vi "144 Swerve Drive 2022.vi"(0 "Joystick X":dbl, 1 "Joystick Y":dbl, 2 "Joystick Z":dbl, 3 "Robot Length(in.)":dbl, 4 "Robot Width(in.)":dbl, 5 "Gyro":dbl, 8 "BL_Steer_Encoder":dbl, 9 "BL PID gains":T1={"proportional gain (Kc)"=0.01, "integral time (Ti, min)"=0.0, "derivative time (Td, min)"=0.0} {"derivative time (Td, min)" format="%.3f"; "integral time (Ti, min)" format="%.3f"; "proportional gain (Kc)" format="%.6f"}, 10 "BR_Steer_Encoder":dbl, 11 "BR PID gains":T1={"proportional gain (Kc)"=0.01, "integral time (Ti, min)"=0.0, "derivative time (Td, min)"=0.0} {"derivative time (Td, min)" format="%.3f"; "integral time (Ti, min)" format="%.3f"; "proportional gain (Kc)" format="%.6f"}, 12 "FL_Steer_Encoder":dbl, 13 "FL PID gains":T1={"proportional gain (Kc)"=0.01, "integral time (Ti, min)"=0.0, "derivative time (Td, min)"=0.0} {"derivative time (Td, min)" format="%.3f"; "integral time (Ti, min)" format="%.3f"; "proportional gain (Kc)" format="%.6f"}, 14 "FR_Steer_Encoder":dbl, 15 "FR PID gains":T1={"proportional gain (Kc)"=0.01, "integral time (Ti, min)"=0.0, "derivative time (Td, min)"=0.0} {"derivative time (Td, min)" format="%.3f"; "integral time (Ti, min)" format="%.3f"; "proportional gain (Kc)" format="%.6f"}) -> (20 "Throttle BL":dbl, 21 "Throttle BR":dbl, 22 "Throttle FL":dbl, 23 "Throttle FR":dbl, 24 "BL_STEER_MOTOR_OUTPUT":dbl, 25 "BR_STEER_MOTOR_OUTPUT":dbl, 26 "FL_STEER_MOTOR_OUTPUT":dbl, 27 "FR_STEER_MOTOR_OUTPUT":dbl)   [LabVIEW 2020]
uses:
  <vilib>/addons/control/pid/pid.llb/PID (DBL).vi
  <vilib>/addons/control/pid/NI_PID_pid.lvlib
panel:
  out "FR_ERROR":dbl
  out "FL_ERROR":dbl
  out "BR_ERROR":dbl
  out "BL_ERROR":dbl
  out "Rotation steering angle BL":dbl
  out "Rotation steering angle FR":dbl
  out "Rotation steering angle FL":dbl
  out "Rotation steering angle BR":dbl
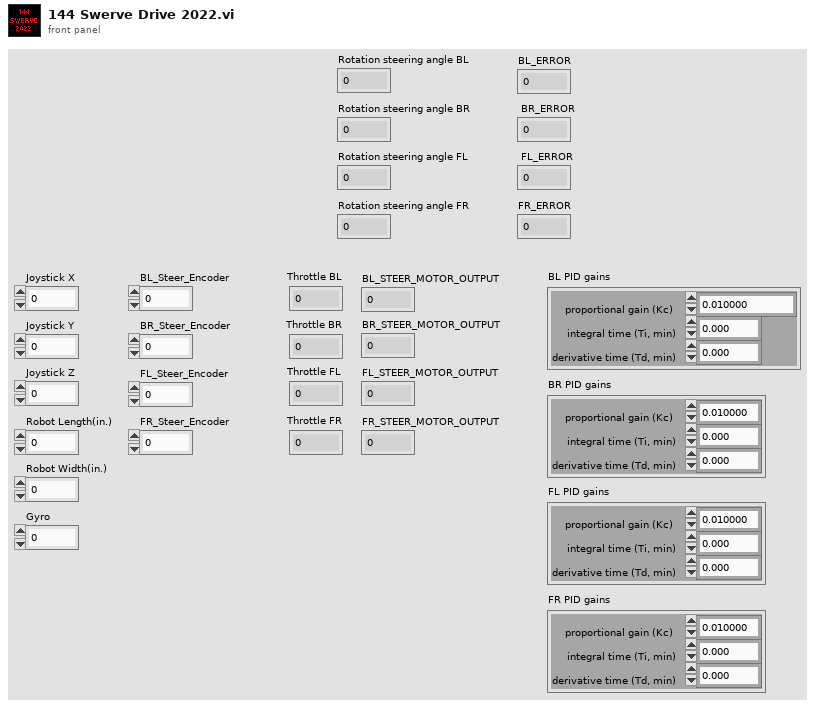
[diagram p1: front panel]
types:
  T1 = cluster{"proportional gain (Kc)":dbl, "integral time (Ti, min)":dbl, "derivative time (Td, min)":dbl}
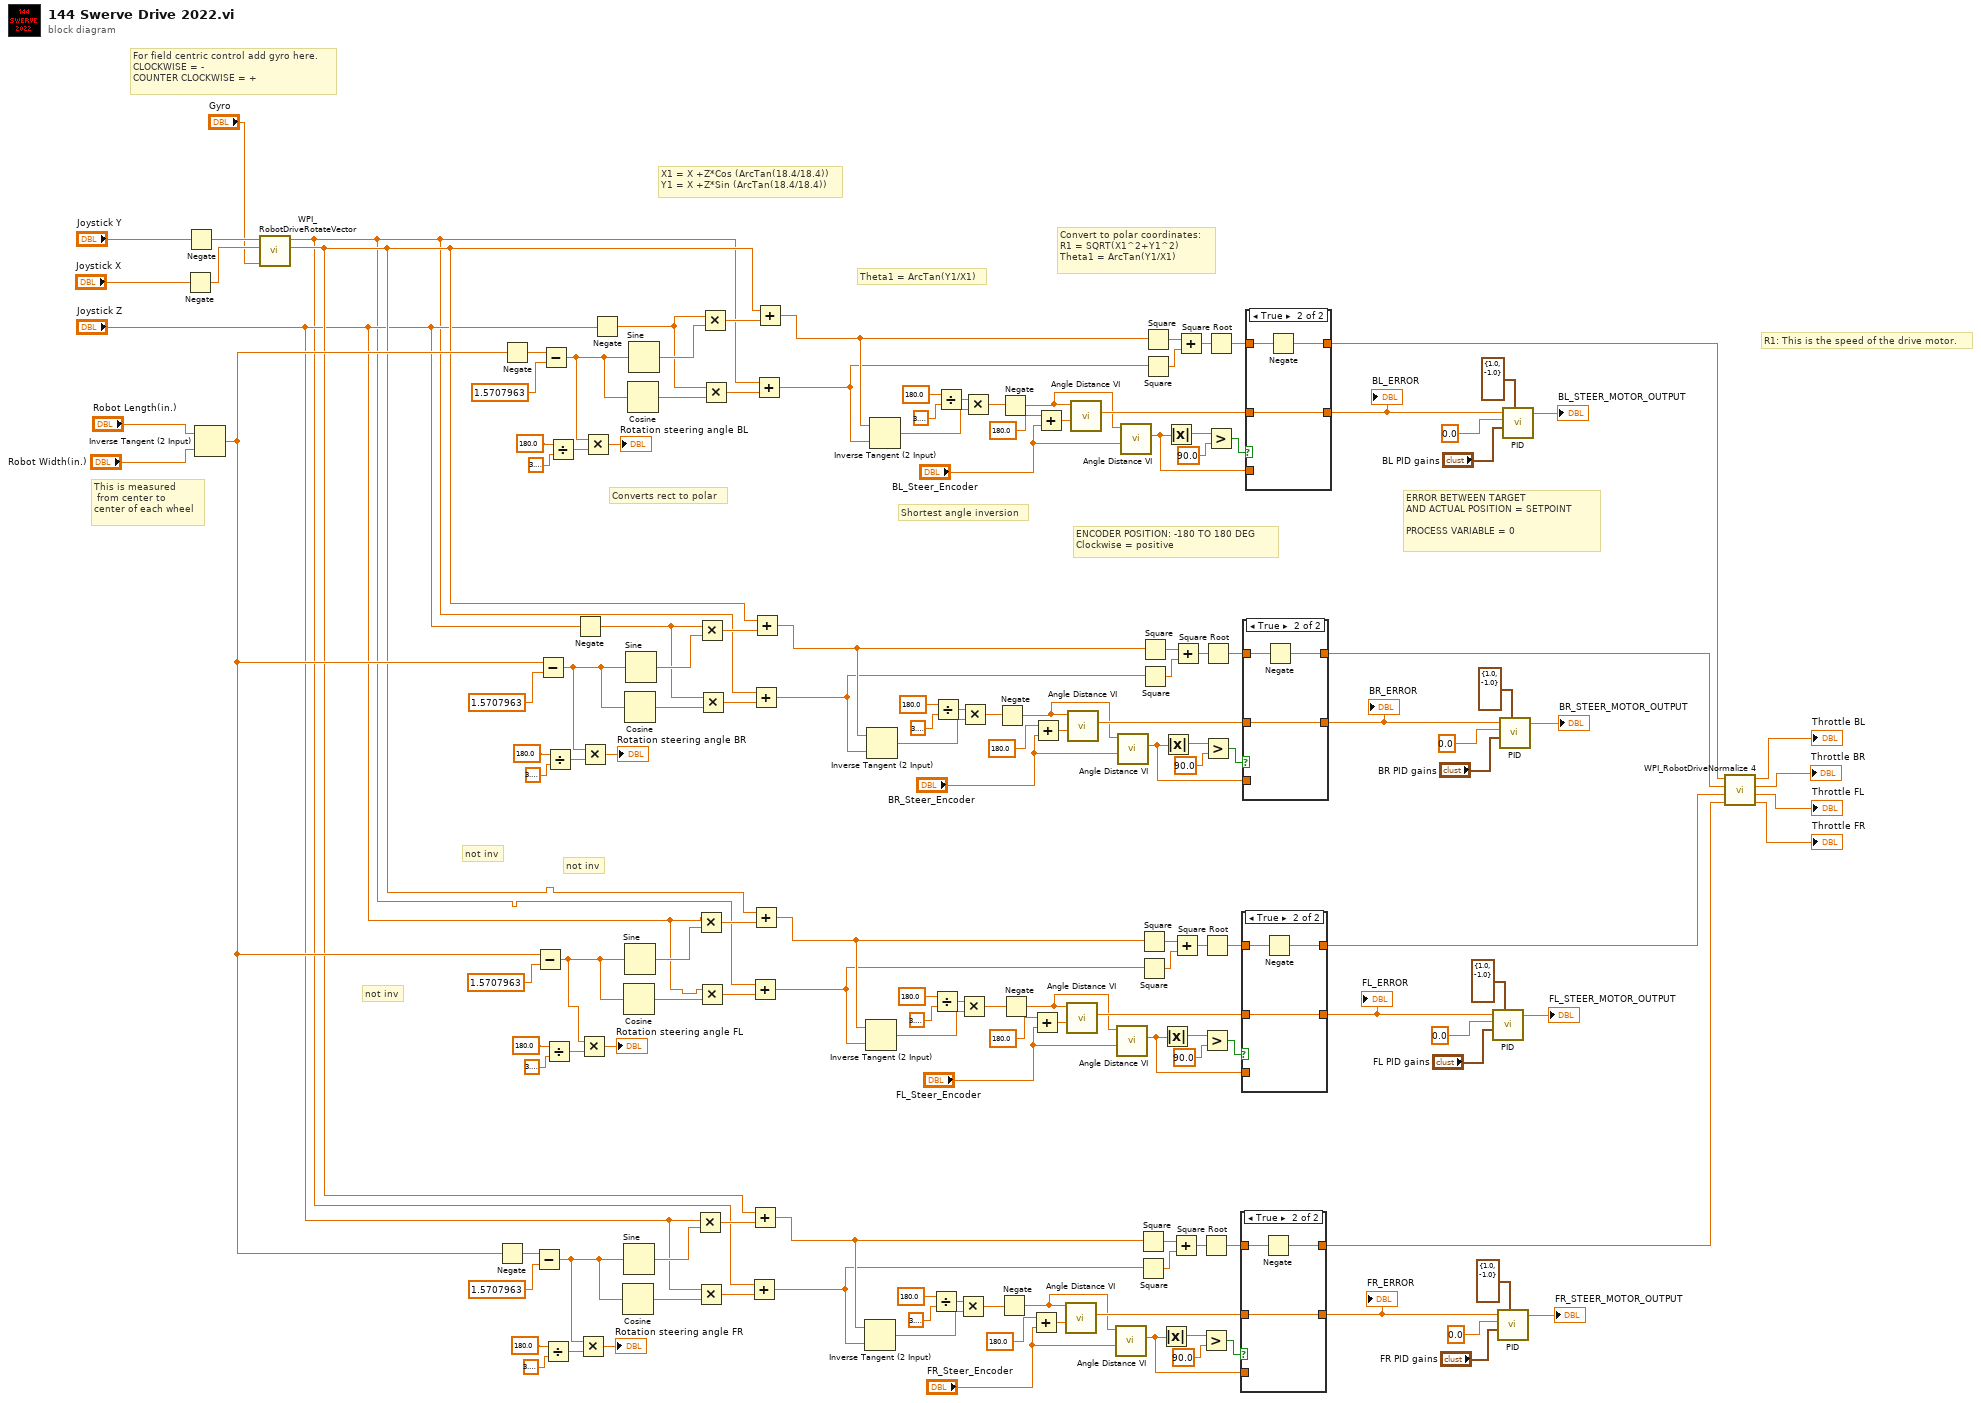
[diagram p0: block diagram]
diagram:
  # "not inv"
  # "not inv"
  # "not inv"
  # "Shortest angle inversion"
  # "Converts rect to polar"
  # "ERROR BETWEEN TARGET\nAND ACTUAL POSITION = SETPOINT\n\nPROCESS VARIABLE = 0"
  # "ENCODER POSITION: -180 TO 180 DEG\nClockwise = positive"
  # "X1 = X +Z*Cos (ArcTan(18.4/18.4))\nY1 = X +Z*Sin (ArcTan(18.4/18.4))"
  # "Theta1 = ArcTan(Y1/X1)"
  # "Convert to polar coordinates:\nR1 = SQRT(X1^2+Y1^2)\nTheta1 = ArcTan(Y1/X1)"
  # "R1: This is the speed of the drive motor."
  # "This is measured\n from center to \ncenter of each wheel"
  # "For field centric control add gyro here.\nCLOCKWISE = -\nCOUNTER CLOCKWISE = +"
  n1 = Negate(x="Joystick X") -> (-x=w163:dbl)
  n2 = Negate(x="Joystick Y") -> (-x=w79:dbl)
  n3 = Inverse Tangent (2 Input)(1:"Robot Width(in.)", 2:"Robot Length(in.)") -> (0:w8:dbl)
  n4 = call <vilib>:"WPI_RobotDriveRotateVector.vi"("Angle"="Gyro", "X"=w163, "Y"=w79) -> ("X'"=w3:dbl, "Y'"=w1:dbl)  [unwired: 7 out]
  n5 = Negate(x=w8) -> (-x=w29:dbl)
  n6 = Negate(x=w8) -> (-x=w44:dbl)
  n7 = Subtract(x=w29, y=1.5707963) -> (x-y=w101:dbl)
  n8 = Subtract(x=w8, y=1.5707963) -> (x-y=w7:dbl)
  n9 = Subtract(x=w8, y=1.5707963) -> (x-y=w77:dbl)
  n10 = Subtract(x=w44, y=1.5707963) -> (x-y=w42:dbl)
  n11 = Divide(x=180.0, y=3.141592653589793) -> (x/y=w100:dbl)
  n12 = Divide(x=180.0, y=3.141592653589793) -> (x/y=w125:dbl)
  n13 = Divide(x=180.0, y=3.141592653589793) -> (x/y=w155:dbl)
  n14 = Divide(x=180.0, y=3.141592653589793) -> (x/y=w67:dbl)
  n15 = Negate(x="Joystick Z") -> (-x=w22:dbl)
  n16 = Multiply(x=w101, y=w100) -> (x*y=→"Rotation steering angle FR":dbl)
  n17 = Multiply(x=w7, y=w125) -> (x*y=→"Rotation steering angle FL":dbl)
  n18 = Multiply(x=w77, y=w155) -> (x*y=→"Rotation steering angle BR":dbl)
  n19 = Multiply(x=w42, y=w67) -> (x*y=→"Rotation steering angle BL":dbl)
  n20 = Negate(x="Joystick Z") -> (-x=w23:dbl)
  n21 = Cosine(x=w101) -> (cos(x)=w96:dbl)
  n22 = Cosine(x=w7) -> (cos(x)=w121:dbl)
  n23 = Sine(x=w101) -> (sin(x)=w95:dbl)
  n24 = Cosine(x=w77) -> (cos(x)=w151:dbl)
  n25 = Sine(x=w7) -> (sin(x)=w120:dbl)
  n26 = Sine(x=w77) -> (sin(x)=w150:dbl)
  n27 = Cosine(x=w42) -> (cos(x)=w63:dbl)
  n28 = Sine(x=w42) -> (sin(x)=w62:dbl)
  n29 = Multiply(x="Joystick Z", y=w95) -> (x*y=w94:dbl)
  n30 = Multiply(x="Joystick Z", y=w120) -> (x*y=w6:dbl)
  n31 = Multiply(x="Joystick Z", y=w96) -> (x*y=w93:dbl)
  n32 = Multiply(x=w22, y=w150) -> (x*y=w149:dbl)
  n33 = Multiply(x="Joystick Z", y=w121) -> (x*y=w119:dbl)
  n34 = Multiply(x=w22, y=w151) -> (x*y=w148:dbl)
  n35 = Multiply(x=w23, y=w62) -> (x*y=w61:dbl)
  n36 = Multiply(x=w23, y=w63) -> (x*y=w60:dbl)
  n37 = Add(x=w1, y=w93) -> (x+y=w91:dbl)
  n38 = Add(x=w1, y=w119) -> (x+y=w117:dbl)
  n39 = Add(x=w3, y=w94) -> (x+y=w92:dbl)
  n40 = Add(x=w1, y=w148) -> (x+y=w146:dbl)
  n41 = Add(x=w3, y=w6) -> (x+y=w118:dbl)
  n42 = Add(x=w3, y=w149) -> (x+y=w147:dbl)
  n43 = Add(x=w1, y=w60) -> (x+y=w58:dbl)
  n44 = Add(x=w3, y=w61) -> (x+y=w59:dbl)
  n45 = Inverse Tangent (2 Input)(1:w91, 2:w92) -> (0:w104:dbl)
  n46 = Inverse Tangent (2 Input)(1:w117, 2:w118) -> (0:w128:dbl)
  n47 = Inverse Tangent (2 Input)(1:w146, 2:w147) -> (0:w158:dbl)
  n48 = Inverse Tangent (2 Input)(1:w58, 2:w59) -> (0:w70:dbl)
  n49 = Divide(x=180.0, y=3.141592653589793) -> (x/y=w105:dbl)
  n50 = Divide(x=180.0, y=3.141592653589793) -> (x/y=w129:dbl)
  n51 = Divide(x=180.0, y=3.141592653589793) -> (x/y=w159:dbl)
  n52 = Divide(x=180.0, y=3.141592653589793) -> (x/y=w71:dbl)
  n53 = Multiply(x=w105, y=w104) -> (x*y=w18:dbl)
  n54 = Multiply(x=w129, y=w128) -> (x*y=w21:dbl)
  n55 = Multiply(x=w159, y=w158) -> (x*y=w76:dbl)
  n56 = Multiply(x=w71, y=w70) -> (x*y=w41:dbl)
  n57 = Negate(x=w76) -> (-x=w75:dbl)
  n58 = Negate(x=w18) -> (-x=w19:dbl)
  n59 = Negate(x=w41) -> (-x=w40:dbl)
  n60 = Negate(x=w21) -> (-x=w20:dbl)
  n61 = Add(x=180.0, y="FR_Steer_Encoder") -> (x+y=w90:dbl)
  n62 = Add(x=180.0, y="FL_Steer_Encoder") -> (x+y=w116:dbl)
  n63 = Add(x=180.0, y="BR_Steer_Encoder") -> (x+y=w145:dbl)
  n64 = Add(x=180.0, y="BL_Steer_Encoder") -> (x+y=w57:dbl)
  n65 = call "Angle Distance VI.vi"("current angle"=w90, "target angle"=w19) -> ("distance"=w85:dbl)  [unwired: 9 in]
  n66 = call "Angle Distance VI.vi"("current angle"=w116, "target angle"=w20) -> ("distance"=w111:dbl)  [unwired: 9 in]
  n67 = call "Angle Distance VI.vi"("current angle"=w145, "target angle"=w75) -> ("distance"=w140:dbl)  [unwired: 9 in]
  n68 = call "Angle Distance VI.vi"("current angle"=w57, "target angle"=w40) -> ("distance"=w52:dbl)  [unwired: 9 in]
  n69 = call "Angle Distance VI.vi"("current angle"="FR_Steer_Encoder", "target angle"=w19) -> ("distance"=w83:dbl)  [unwired: 9 in]
  n70 = call "Angle Distance VI.vi"("current angle"="FL_Steer_Encoder", "target angle"=w20) -> ("distance"=w109:dbl)  [unwired: 9 in]
  n71 = call "Angle Distance VI.vi"("current angle"="BR_Steer_Encoder", "target angle"=w75) -> ("distance"=w138:dbl)  [unwired: 9 in]
  n72 = call "Angle Distance VI.vi"("current angle"="BL_Steer_Encoder", "target angle"=w40) -> ("distance"=w50:dbl)  [unwired: 9 in]
  n73 = Square(x=w92) -> (x^2=w108:dbl)
  n74 = Square(x=w91) -> (x^2=w106:dbl)
  n75 = Square(x=w118) -> (x^2=w132:dbl)
  n76 = Square(x=w117) -> (x^2=w130:dbl)
  n77 = Square(x=w147) -> (x^2=w162:dbl)
  n78 = Square(x=w146) -> (x^2=w160:dbl)
  n79 = Square(x=w59) -> (x^2=w74:dbl)
  n80 = Square(x=w58) -> (x^2=w72:dbl)
  n81 = Absolute Value(x=w83) -> (abs(x)=w87:dbl)
  n82 = Absolute Value(x=w109) -> (abs(x)=w113:dbl)
  n83 = Absolute Value(x=w138) -> (abs(x)=w142:dbl)
  n84 = Absolute Value(x=w50) -> (abs(x)=w54:dbl)
  n85 = Add(x=w108, y=w106) -> (x+y=w107:dbl)
  n86 = Add(x=w132, y=w130) -> (x+y=w131:dbl)
  n87 = Add(x=w162, y=w160) -> (x+y=w161:dbl)
  n88 = Add(x=w74, y=w72) -> (x+y=w73:dbl)
  n89 = Square Root(x=w107) -> (sqrt(x)=w84:dbl)
  n90 = Greater?(x=w87, y=90.0 ("x")) -> (0:w88:bool)
  n91 = Square Root(x=w131) -> (sqrt(x)=w110:dbl)
  n92 = Greater?(x=w113, y=90.0 ("x")) -> (0:w114:bool)
  n93 = Square Root(x=w161) -> (sqrt(x)=w139:dbl)
  n94 = Greater?(x=w142, y=90.0 ("x")) -> (0:w143:bool)
  n95 = Square Root(x=w73) -> (sqrt(x)=w51:dbl)
  n96 = Greater?(x=w54, y=90.0 ("x")) -> (0:w55:bool)
  n97 = case shown="True" w88 {
    tunnel: w83 -> [w165 _]
    tunnel: [w165 w168] -> w82
    tunnel: w85 -> [_ w168]
    tunnel: w84 -> [w164 w167]
    tunnel: [w164 w166] -> w80
    frame False {
    }
    frame True {
      n98 = Negate(x=w167) -> (-x=w166:dbl)
    }
  }
  "FR_ERROR" <- w82
  n99 = case shown="True" w114 {
    tunnel: w109 -> [w170 _]
    tunnel: [w170 w173] -> w31
    tunnel: w111 -> [_ w173]
    tunnel: w110 -> [w169 w172]
    tunnel: [w169 w171] -> w81
    frame False {
    }
    frame True {
      n100 = Negate(x=w172) -> (-x=w171:dbl)
    }
  }
  "FL_ERROR" <- w31
  n101 = case shown="True" w143 {
    tunnel: w138 -> [w175 _]
    tunnel: [w175 w178] -> w135
    tunnel: w140 -> [_ w178]
    tunnel: w139 -> [w174 w177]
    tunnel: [w174 w176] -> w137
    frame False {
    }
    frame True {
      n102 = Negate(x=w177) -> (-x=w176:dbl)
    }
  }
  "BR_ERROR" <- w135
  n103 = case shown="True" w55 {
    tunnel: w50 -> [w180 _]
    tunnel: [w180 w183] -> w49
    tunnel: w52 -> [_ w183]
    tunnel: w51 -> [w179 w182]
    tunnel: [w179 w181] -> w39
    frame False {
    }
    frame True {
      n104 = Negate(x=w182) -> (-x=w181:dbl)
    }
  }
  "BL_ERROR" <- w49
  n105 = call-poly <vilib>:"PID.vi"("output range"=cluster{"output high":dbl, "output low":dbl} {"output high"=1.0, "output low"=-1.0}, "PID gains"="FL PID gains", "process variable"=0.0, "setpoint"=w31) -> ("output"=→"FL_STEER_MOTOR_OUTPUT":dbl)  [unwired: 6 in, 1 out]
  n106 = call-poly <vilib>:"PID.vi"("output range"=cluster{"output high":dbl, "output low":dbl} {"output high"=1.0, "output low"=-1.0}, "PID gains"="FR PID gains", "process variable"=0.0, "setpoint"=w82) -> ("output"=→"FR_STEER_MOTOR_OUTPUT":dbl)  [unwired: 6 in, 1 out]
  n107 = call-poly <vilib>:"PID.vi"("output range"=cluster{"output high":dbl, "output low":dbl} {"output high"=1.0, "output low"=-1.0}, "PID gains"="BR PID gains", "process variable"=0.0, "setpoint"=w135) -> ("output"=→"BR_STEER_MOTOR_OUTPUT":dbl)  [unwired: 6 in, 1 out]
  n108 = call-poly <vilib>:"PID.vi"("output range"=cluster{"output high":dbl, "output low":dbl} {"output high"=1.0, "output low"=-1.0}, "PID gains"="BL PID gains", "process variable"=0.0, "setpoint"=w49) -> ("output"=→"BL_STEER_MOTOR_OUTPUT":dbl)  [unwired: 6 in, 1 out]
  n109 = call <vilib>:"WPI_RobotDriveNormalize 4.vi"("D"=w80, "C"=w81, "B"=w137, "A"=w39) -> ("D'"=→"Throttle FR":dbl, "C'"=→"Throttle FL":dbl, "B'"=→"Throttle BR":dbl, "A'"=→"Throttle BL":dbl)
